vi "Set Channel Voltage.vi"(8 "error in (no error)":errorcluster, 9 "Channel Select":enum16{"Channel 1", "Channel 2", "Channel 3"}(ring), 10 "Voltage":dbl format="%#_13g", 11 "2230G in":refnum<class "2230G.lvclass">) -> (0 "error out":errorcluster, 3 "2230G out":refnum<class "2230G.lvclass">)   [LabVIEW 2018, in "2230G.lvlib" / "2230G.lvclass"]
uses:
  2230G.lvclass
  PPLs/Power Supply/Parent/Power_Supply.lvlibp/Custom Control/Protection.ctl
  2230G.lvclass/2230G.ctl
  PPLs/Power Supply/Parent/Power_Supply.lvlibp/Power Supply.lvclass
  <instrlib>/Keithley KE22xx Series/Keithley KE22xx Series.lvlib
  PPLs/Power Supply/Parent/Power_Supply.lvlibp
  C:/Projects/LabVIEW/PPLs/Power Supply/Parent/Power_Supply.lvlibp/Power Supply.lvclass
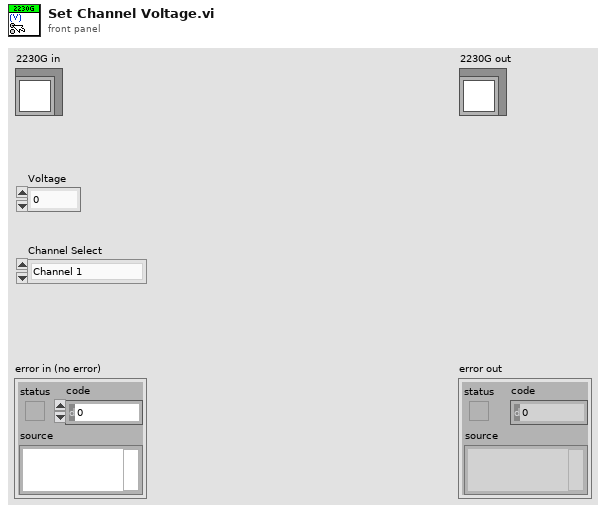
[diagram p1: front panel]
types:
  T1 = typedef "Power_Supply.lvlibp/Protection.ctl" = enum16{"None", "Over Volt", "Under Volt", "Over Current"}
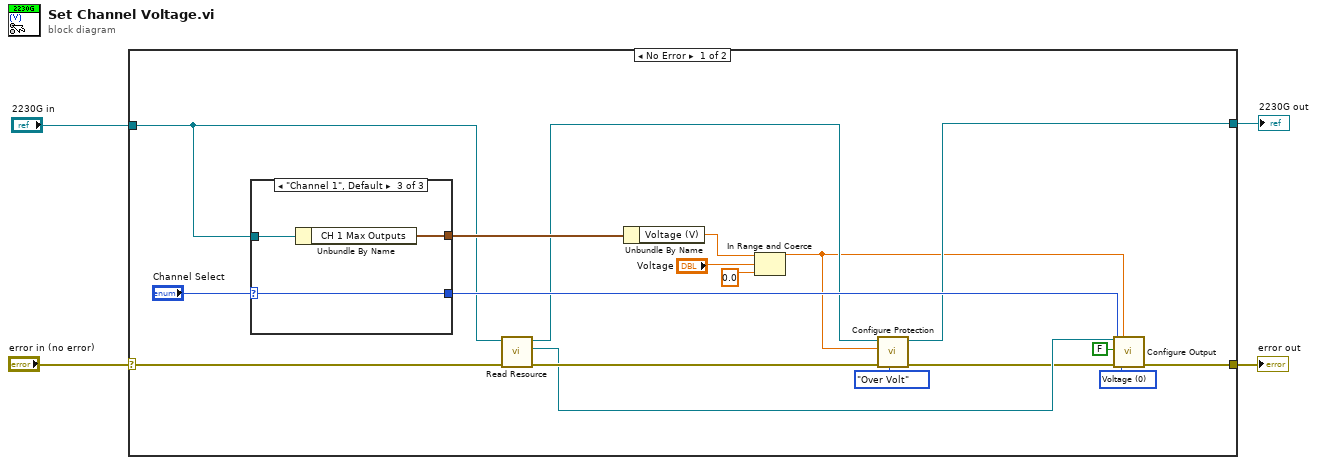
[diagram p0: block diagram]
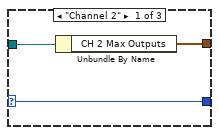
[diagram p2: hidden frame]
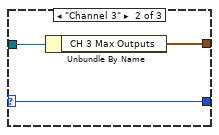
[diagram p3: hidden frame]
diagram:
  n1 = case shown="No Error" "error in (no error)" {
    selector: "error in (no error)" -> [w13 w33]
    tunnel: [w6 w33] -> w3
    tunnel: [w11 w32] -> w1
    tunnel: "2230G in" -> [w14 w32]
    frame No Error {
      w17 = u16 0 items=["Voltage", "Current"] ("Function(0:Voltage)")
      n2 = case shown="\"Channel 1\", Default" "Channel Select" {
        selector: "Channel Select" -> [w23 w26 w29]
        tunnel: w14 -> [w25 w27 w31]
        tunnel: [w24 w28 w30] -> w21
        tunnel: [w23 w26 w29] -> w15
        frame "Channel 2" {
          n3 = Unbundle By Name(w25) -> ("CH 2 Max Outputs"=w24:cluster{"Voltage (V)":dbl, "Current (A)":dbl})
        }
        frame "Channel 3" {
          n4 = Unbundle By Name(w27) -> ("CH 3 Max Outputs"=w28:cluster{"Voltage (V)":dbl, "Current (A)":dbl})
        }
        frame "Channel 1", Default {
          n5 = Unbundle By Name(w31) -> ("CH 1 Max Outputs"=w30:cluster{"Voltage (V)":dbl, "Current (A)":dbl})
        }
      }
      n6 = call "Read Resource.vi"("error in"=w13, "Power Supply in"=w14) -> ("error out"=w9:errorcluster, "Resource"=w8:refnum<visa-resource-name>, "Power Supply out"=w12:refnum<class "2230G.lvclass">)  [unwired: 7 in]
      n7 = Unbundle By Name(w21) -> ("Voltage (V)"=w20:dbl)
      n8 = In Range and Coerce(upper limit=w20, x="Voltage", lower limit=0.0) -> (coerced(x)=w5:dbl)  [unwired: 1 out]
      n9 = call-dynamic "Configure Protection.vi"("Protection (None)"=Protection."Over Volt", "error in (no error)"=w9, "Limit"=w5, "2230G in"=w12) -> ("error out"=w7:errorcluster, "2230G out"=w11:refnum<class "2230G.lvclass">)  [unwired: 6 in]
      n10 = call <instrlib>:"Configure Output.vi"("VISA resource name"=w8, "Manual Range(0.00)"=w5, "Channel Select"=w15, "Function(0:Voltage)"=w17, "Enable Output (T: Enable)"=FALSE, "error in (no error)"=w7) -> ("error out"=w6:errorcluster)  [unwired: 8 in, 1 out]
    }
    frame Error {
    }
  }
  "error out" <- w3
  "2230G out" <- w1
